vi "Set Cursor Pos.vi"(7 "lpPoint":cluster{"X":i32, "Y":i32}) -> ()   [LabVIEW 2011]
uses:
  USER32.DLL
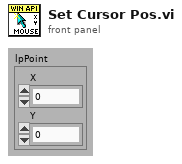
[diagram p1: front panel]
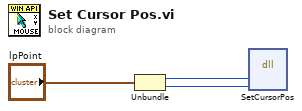
[diagram p0: block diagram]
diagram:
  n1 = Unbundle("lpPoint") -> ("X"=w2:i32, "Y"=w1:i32)
  n2 = dll-call lib="user32.dll" fn="SetCursorPos"("X"=w2, "Y"=w1) -> ()  [unwired: 6 in, 2 out]
